vi "00 Main (three phase) (x64-2018).vi"() -> ()   [LabVIEW 2017]
uses:
  <vilib>/DAQmx/read.llb/DAQmx Read (Analog 1D Wfm NChan NSamp).vi
  <vilib>/DAQmx/miscellaneous.llb/DAQmx Fill In Error Info.vi
panel:
  out "Error Out":errorcluster
  out "Waveform Graph":waveform(dbl)[](graph)
  in  "DAQmx Task Name":refnum<k21>
  out "Error out (DAQ Loop)":errorcluster
  out "DAQ Loop Iterations":i32
  out "Raw DAQ Output":dynamicdata(graph)=[{"t0"=timestamp(3367839419.335167 s since 1904-01-01), "dt"=0.00016666666666666663, "Y"=array[240 elements], "attributes"=variant("NI_ChannelName"=variant(string "Voltage_0"), "NI_UnitDescription"=variant(string "Volts"))}, {"t0"=timestamp(3367839419.3351874 s since 1904-01-01), "dt"=0.00016666666666666663, "Y"=array[240 elements], "attributes"=variant("NI_ChannelName"=variant(string "Voltage_1"), "NI_UnitDescription"=variant(string "Volts"))}, {"t0"=timestamp(3367839419.3352084 s since 1904-01-01), "dt"=0.00016666666666666663, "Y"=array[240 elements], "attributes"=variant("NI_ChannelName"=variant(string "Voltage_2"), "NI_UnitDescription"=variant(string "Volts"))}]
  in  "All Stop!":bool
  out "Frequency 2":dynamicdata(graph)=[{"t0"=timestamp(3424329819.6880417 s since 1904-01-01), "dt"=0.00016666666666666663, "Y"=[50.00644377121546], "attributes"=variant("NI_ChannelName"=variant(string "Detected Frequency"))}, {"t0"=timestamp(3424329819.6880627 s since 1904-01-01), "dt"=0.00016666666666666663, "Y"=[49.993846178541475], "attributes"=variant("NI_ChannelName"=variant(string "Detected Frequency"))}, {"t0"=timestamp(3424329819.6880836 s since 1904-01-01), "dt"=0.00016666666666666663, "Y"=[49.994041382621866], "attributes"=variant("NI_ChannelName"=variant(string "Detected Frequency"))}] caption="Frequency"
  out "Phase 2":dynamicdata(graph)=[{"t0"=timestamp(3424329819.6880417 s since 1904-01-01), "dt"=0.00016666666666666663, "Y"=[-19.090260250465658], "attributes"=variant("NI_ChannelName"=variant(string "Detected Phase"))}, {"t0"=timestamp(3424329819.6880627 s since 1904-01-01), "dt"=0.00016666666666666663, "Y"=[-138.45601955575555], "attributes"=variant("NI_ChannelName"=variant(string "Detected Phase"))}, {"t0"=timestamp(3424329819.6880836 s since 1904-01-01), "dt"=0.00016666666666666663, "Y"=[102.37498697247455], "attributes"=variant("NI_ChannelName"=variant(string "Detected Phase"))}] caption="Frequency"
  out "Frequency":dbl format="%.2f"
  out "Amplitude":dbl format="%.2f"
  out "Phase":dbl format="%.2f"
  out "Acquisition Time":timestamp
  out "Voltage Waveform":dynamicdata(graph)=[{"t0"=timestamp(3424329819.638042 s since 1904-01-01), "dt"=0.00016666666666666663, "Y"=array[300 elements]}, {"t0"=timestamp(3424329819.6380625 s since 1904-01-01), "dt"=0.00016666666666666663, "Y"=array[300 elements]}, {"t0"=timestamp(3424329819.6380835 s since 1904-01-01), "dt"=0.00016666666666666663, "Y"=array[300 elements]}]
  out "IP":string
  out "Port":i32
  out "Transmitted Data":string
  out "Stop":bool
  out "Elements in Acquisition Buffer":i32
  # "V1.2 - PFI0 (Three Phase)"
  # "50.5"
  # "49.5"
  # "The code and design of this VI are licensed \nunder the terms of the New BSD License.\nPlease see the VI documentation or License.txt\nfor more details.\n\nCopyright (c) 2012, David Laverty\nwww.OpenPMU.org"
  # "180"
  # "-180"
  # "Configuration Information:\n\nThe ID and IP address to which the OpenPMU sends data is configured by 'C:\\PMUconfig.ini'.  If this doesn't exist, create it.\n\nCopy and paste the blue text below without the dashed lines into PMUconfig.ini.\n\n[Telecoms]\nID=PMU123\nIP=192.168.1.100\nPort=40001\n\nIP and Port may be any values within normal IPv4 range.  ID should be six alpha-numeric characters."
  # "Debug Stuff ( you're not supposed to find this :P )"
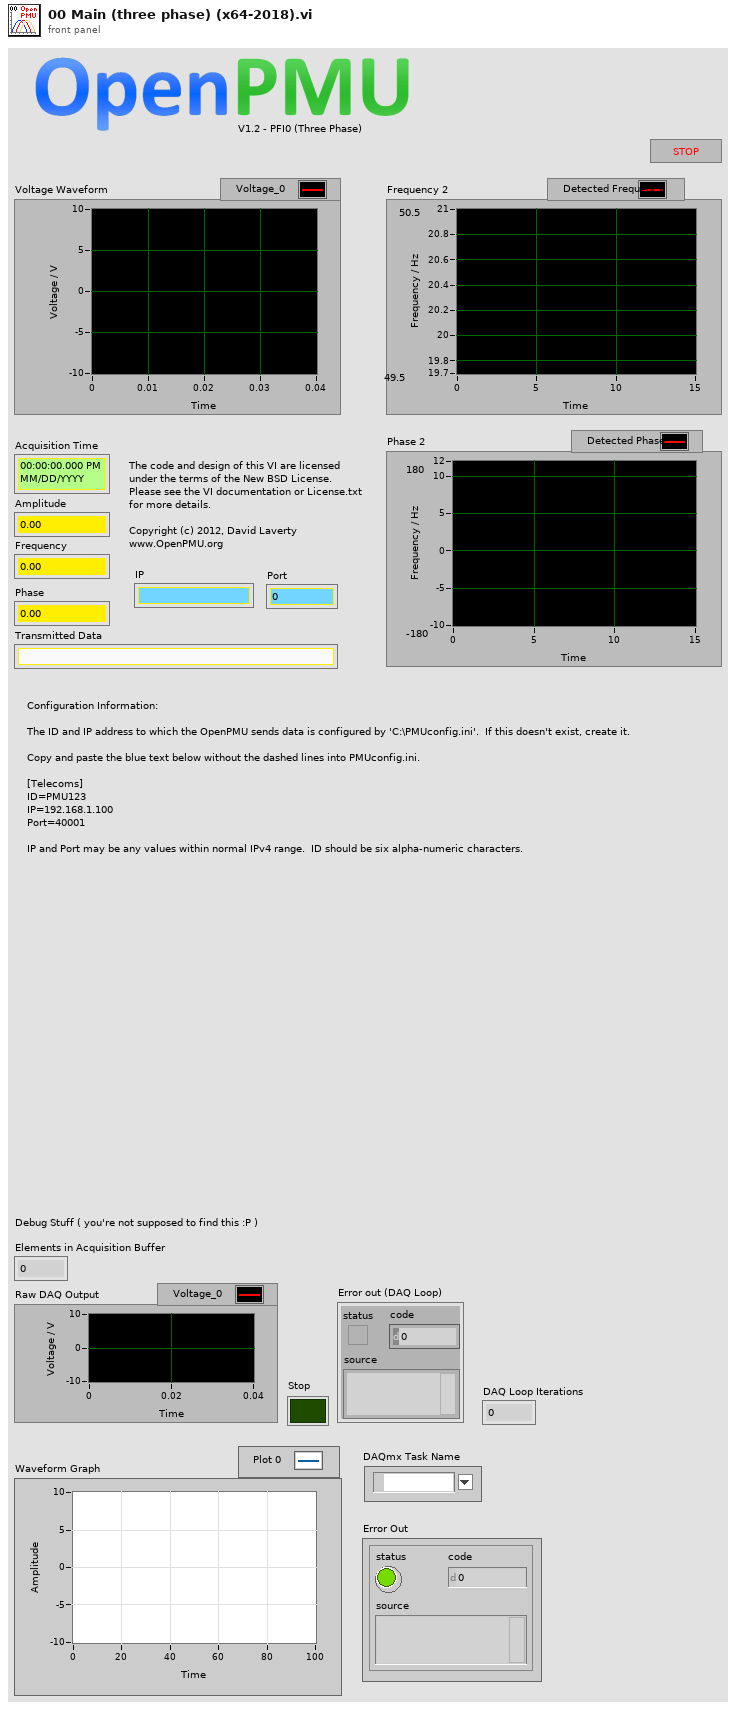
[diagram p1: front panel]
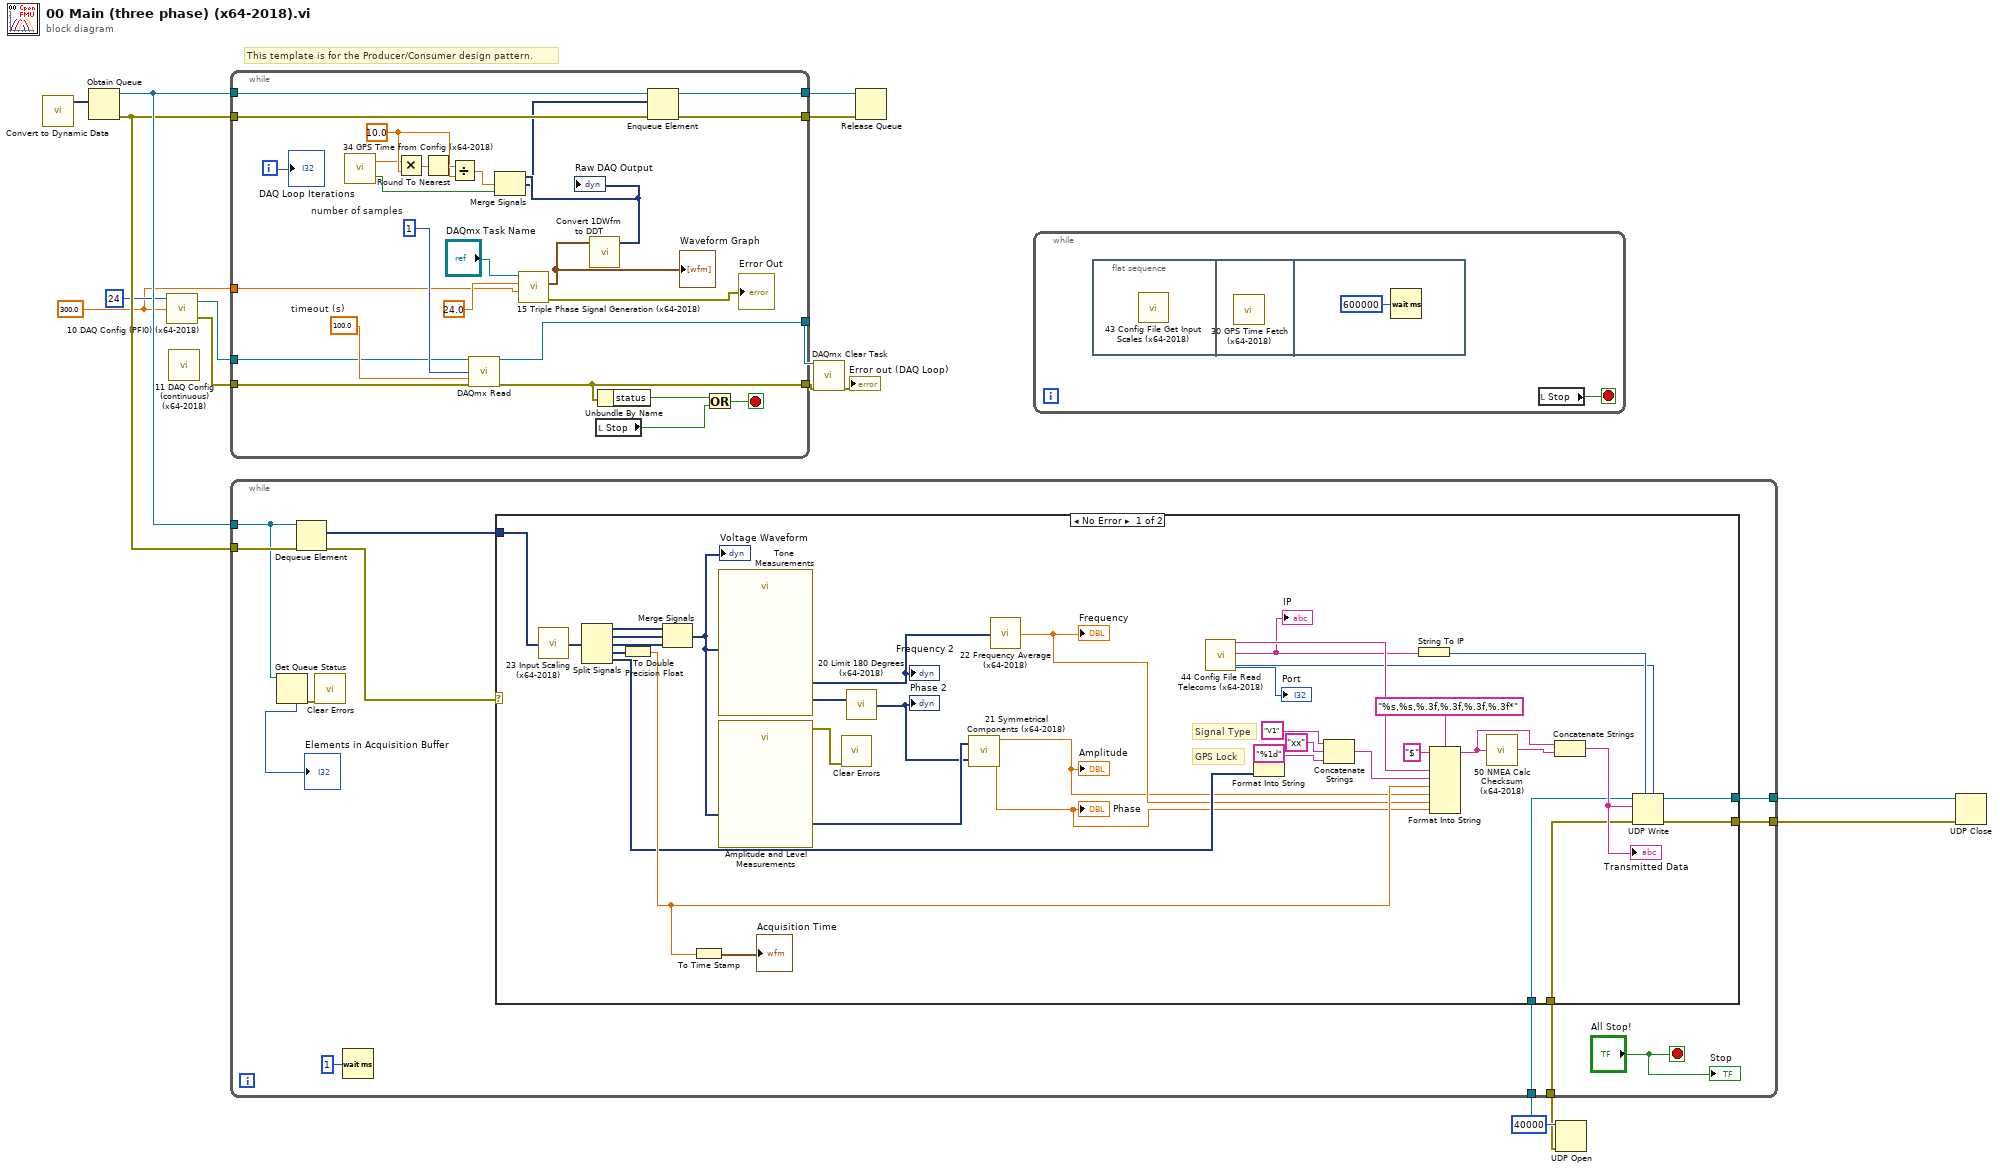
[diagram p0: block diagram]
diagram:
  w1 = 300.0 ("rate")
  # "This template is for the Producer/Consumer design pattern."
  n1 = call "Convert to Dynamic Data"() -> ("Dynamic Data Type"=w14:dynamicdata)  [unwired: 4 in]
  n2 = Obtain Queue(element data type=w14) -> (queue out=w11:refnum<queue>, error out=w10:errorcluster)  [unwired: 4 in, 1 out]
  n3 = call "10 DAQ Config (PFI0) (x64-2018).vi"("rate"=w1, "number of samples"=24) -> ("Error Out"=w2:errorcluster, "task out"=w3:refnum<k21>)  [unwired: 1 in]
  n4 = call "11 DAQ Config (continuous) (x64-2018).vi"() -> ()  [unwired: 1 in, 2 out]
  n5 = while {
    tunnel: w2 -> [w31]
    tunnel: w3 -> [w32]
    tunnel: [w41] -> w17
    tunnel: [w40] -> w16
    tunnel: w11 -> [w36]
    tunnel: w10 -> [w35]
    tunnel: [w34] -> w13
    tunnel: [w33] -> w12
    tunnel: w1 -> [w20]
    i -> [w39]
    stop <- w38 stop-if-true
    w25 = 10.0 ("y")
    w42 = 100.0  # timeout (s)
    w44 = 1  # number of samples
    n6 = call "34 GPS Time from Config (x64-2018).vi"() -> ("GPS Lock"=w23:bool, "Time"=w24:dbl)  [unwired: 2 in]
    n7 = Multiply(x=w24, y=w25) -> (x*y=w28:dbl)
    n8 = Round To Nearest(number=w28) -> (nearest integer value=w27:dbl)
    n9 = Divide(x=w27, y=w25) -> (x/y=w26:dbl)
    n10 = call-poly <vilib>:"DAQmx Read.vi"("task/channels in"=w32, "number of samples per channel"=w44, "timeout"=w42, "error in"=w31) -> ("task out"=w41:refnum<k21>, "error out"=w40:errorcluster)  [unwired: 9 in, 1 out]
    n11 = call "15 Triple Phase Signal Generation (x64-2018).vi"("Rate"=w20, "Number of samples per channel"=24.0 ("rate"), "task/channels in"="DAQmx Task Name") -> ("Error Out"=→"Error Out":errorcluster, "data"=w19:waveform(dbl)[])  [unwired: 6 in, 1 out]
    "Waveform Graph" <- w19
    n12 = call <vilib>:"Convert 1DWfm to DDT.vi"("Array of Waveforms"=w19) -> ("Dynamic Data Type"=w30:dynamicdata)  [unwired: 3 in]
    "Raw DAQ Output" <- w30
    n13 = Merge Signals(w30, w26, w23) -> (w29:dynamicdata)
    n14 = local read "Stop"() -> (w37:bool)
    n15 = Unbundle By Name(w40) -> ("status"=w43:bool)
    n16 = Enqueue Element(queue=w36, element=w29, error in (no error)=w35) -> (queue out=w34:refnum<queue>, error out=w33:errorcluster)  [unwired: 1 in, 1 out]
    n17 = Or(x=w43, y=w37) -> (x .or. y?=w38:bool)
    "DAQ Loop Iterations" <- w39
  }
  n18 = call <vilib>:"DAQmx Clear Task.vi"("task in"=w17, "error in"=w16) -> ("error out"=→"Error out (DAQ Loop)":errorcluster)  [unwired: 13 in]
  n19 = Release Queue(queue=w13, error in (no error)=w12) -> ()  [unwired: 1 in, 3 out]
  n20 = while {
    stop <- w45 stop-if-true
    n21 = flat-sequence {
      frame #0 {
        n22 = call "43 Config File Get Input Scales (x64-2018).vi"() -> ()  [unwired: 1 in]
      }
      frame #1 {
        n23 = call "30 GPS Time Fetch (x64-2018).vi"() -> ()  [unwired: 1 in]
      }
      frame #2 {
        n24 = Wait (ms)(milliseconds to wait=u32 600000) -> ()  [unwired: 1 out]
      }
    }
    n25 = local read "Stop"() -> (w45:bool)
  }
  n26 = UDP Open(11:u16 40000 ("port")) -> (port=w8:refnum<k16>, 0:w7:errorcluster)  [unwired: 4 in, 1 out]
  n27 = while {
    tunnel: w11 -> [w52]
    tunnel: w10 -> [w54]
    tunnel: w8 -> [w51]
    tunnel: w7 -> [w50]
    tunnel: [w49] -> w6
    tunnel: [w48] -> w5
    stop <- "All Stop!" stop-if-true
    n28 = Get Queue Status(queue=w52) -> (error out=w47:errorcluster, # elements in queue=→"Elements in Acquisition Buffer":i32)  [unwired: 2 in, 6 out]
    n29 = Dequeue Element(queue=w52, error in (no error)=w54) -> (element=w55:dynamicdata, error out=w56:errorcluster)  [unwired: 1 in, 2 out]
    n30 = call <vilib>:"Clear Errors.vi"("error in (no error)"=w47) -> ()  [unwired: 5 in, 2 out]
    n31 = Wait (ms)(milliseconds to wait=u32 1) -> ()  [unwired: 1 out]
    n32 = case shown="No Error" w56 {
      tunnel: w55 -> [w60 _]
      tunnel: w51 -> [w88 w96]
      tunnel: w50 -> [w87 w95]
      tunnel: [w86 w96] -> w49
      tunnel: [w85 w95] -> w48
      frame No Error {
        # "GPS Lock"
        # "Signal Type"
        n33 = call "23 Input Scaling (x64-2018).vi"("Input (Raw)"=w60) -> ("Output (Scaled)"=w59:dynamicdata)
        n34 = Split Signals(w59) -> (w73:dynamicdata, w74:dynamicdata, w75:dynamicdata, w84:dynamicdata, w82:dynamicdata)  [unwired: 5 in]
        n35 = To Double Precision Float(number=w84) -> (double precision float=w83:dbl)
        n36 = Merge Signals(w73, w74, w75) -> (w76:dynamicdata)
        "Voltage Waveform" <- w76
        n37 = To Time Stamp(1:w83) -> (0:→"Acquisition Time":timestamp)
        n38 = call "Tone Measurements"("Signals"=w76) -> ("Phase"=w72:dynamicdata, "Frequency"=w71:dynamicdata)  [unwired: 7 in, 2 out]
        "Frequency 2" <- w71
        n39 = call "Amplitude and Level Measurements"("Signals"=w76) -> ("Cycle RMS"=w69:dynamicdata, "error out"=w94:errorcluster)  [unwired: 13 in]
        n40 = call <vilib>:"Clear Errors.vi"("error in (no error)"=w94) -> ()  [unwired: 5 in, 2 out]
        n41 = call "20 Limit 180 Degrees (x64-2018).vi"("Angle In"=w72) -> ("Angle Out"=w68:dynamicdata)
        "Phase 2" <- w68
        n42 = call "21 Symmetrical Components (x64-2018).vi"("Amplitude"=w69, "Phase"=w68) -> ("V1"=w67:dbl, "Theta1"=w66:dbl)  [unwired: 4 out]
        "Amplitude" <- w67
        "Phase" <- w66
        n43 = call "22 Frequency Average (x64-2018).vi"("Frequency"=w71) -> ("Numeric"=w70:dbl)
        "Frequency" <- w70
        n44 = call "44 Config File Read Telecoms (x64-2018).vi"() -> ("Port"=w61:i32, "IP"=w62:string, "ID"=w63:string)  [unwired: 3 in]
        "IP" <- w62
        "Port" <- w61
        n45 = Format Into String(format string="%1d", w82) -> (resulting string=w77:string)  [unwired: 2 in, 1 out]
        n46 = Concatenate Strings("V1" ("input 2"), "xx" ("string"), w77) -> (w79:string)
        n47 = String To IP(1:w62) -> (0:w90:u32)
        n48 = Format Into String(format string="%s,%s,%.3f,%.3f,%.3f,%.3f*", initial string="$", w63, w79, w83, w67, w70, w66) -> (resulting string=w65:string)  [unwired: 1 in, 1 out]
        n49 = call "50 NMEA Calc Checksum (x64-2018).vi"("GPS String"=w65) -> ("hex integer string"=w64:string)  [unwired: 1 in, 1 out]
        n50 = Concatenate Strings(w65, w64) -> (w89:string)
        "Transmitted Data" <- w89
        n51 = UDP Write(address=w90, port or service name=w61, connection ID=w88, data in=w89, 8:w87) -> (error out=w85:errorcluster, 3:w86:refnum<k16>)  [unwired: 1 in]
      }
      frame Error {
      }
    }
    "Stop" <- "All Stop!"
  }
  n52 = UDP Close(connection ID=w6, 8:w5) -> ()  [unwired: 2 out]
